vi "Get Debug and Sim.vi"(8 "error in (no error)":errorcluster, 11 "Base Path":path) -> (0 "error out":errorcluster, 3 "Sim + Debug":T1)   [LabVIEW 2012, in "FileIO lib.lvlib"]
doc: "Sets the debug and sim plafs if a file named SIMULATE.txt or DEBUG.txt is found at the source path."
uses:
  FileIO lib.lvlib
  Debug and Sim Flag cluster.ctl
  Project Vis/Globals/Misc static globals.vi
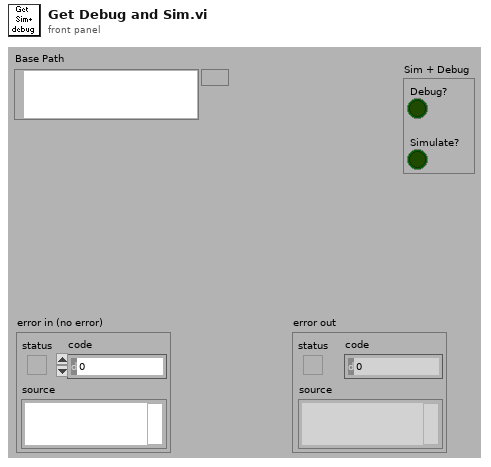
[diagram p1: front panel]
types:
  T1 = typedef "FileIO lib.lvlib/Debug and Sim Flag cluster.ctl" = cluster{"Debug?":bool, "Simulate?":bool}
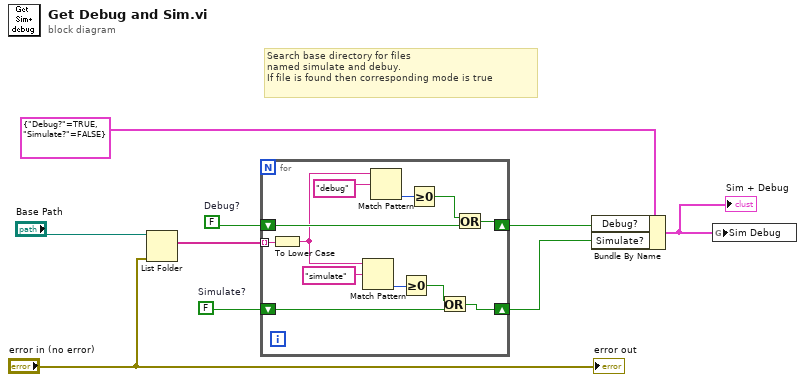
[diagram p0: block diagram]
diagram:
  w4 = FALSE  # Simulate?
  w5 = FALSE  # Debug?
  # "Search base directory for files\nnamed simulate and debuy.\nIf file is found then corresponding mode is true"
  n1 = List Folder(path="Base Path", error in="error in (no error)") -> (filenames=w6:string[])  [unwired: 5 out]
  n2 = for {
    tunnel: w6 -> [w11] mode=indexing
    shift-right: [w18] -> w2
    shift-left: w5 -> [w19]
    shift-right: [w16] -> w3
    shift-left: w4 -> [w17]
    n3 = To Lower Case(string=w11) -> (all lower case string=w10:string)
    n4 = Match Pattern(string=w10, regular expression="simulate") -> (offset past match=w15:i32)  [unwired: 4 out]
    n5 = Match Pattern(string=w10, regular expression="debug") -> (offset past match=w13:i32)  [unwired: 4 out]
    n6 = Greater Or Equal To 0?(x=w15) -> (x >= 0?=w14:bool)
    n7 = Greater Or Equal To 0?(x=w13) -> (x >= 0?=w12:bool)
    n8 = Or(x=w14, y=w17) -> (x .or. y?=w16:bool)
    n9 = Or(x=w12, y=w19) -> (x .or. y?=w18:bool)
  }
  n10 = Bundle By Name(cluster=cluster{"Debug?":bool, "Simulate?":bool} {"Debug?"=TRUE, "Simulate?"=FALSE}, "Debug?"=w2, "Simulate?"=w3) -> (w1:cluster{"Debug?":bool, "Simulate?":bool})
  "Sim + Debug" <- w1
  n11 = global write "Misc static globals.vi" "Sim Debug"(w1) -> ()
  "error out" <- "error in (no error)"
